vi "zad1.vi"() -> ()   [LabVIEW 2017]
panel:
  out "XY Graph":cluster{"Array":dbl[], dbl[]}(graph)
  out "error out":errorcluster
  in  "error in (no error)":errorcluster
  in  "Zakres":cluster{"Min":dbl, "Max":dbl, "Krok":dbl}
  in  "Wspo³czynniki wielomianu":cluster{"a":dbl, "b":dbl, "c":dbl, "d":dbl}
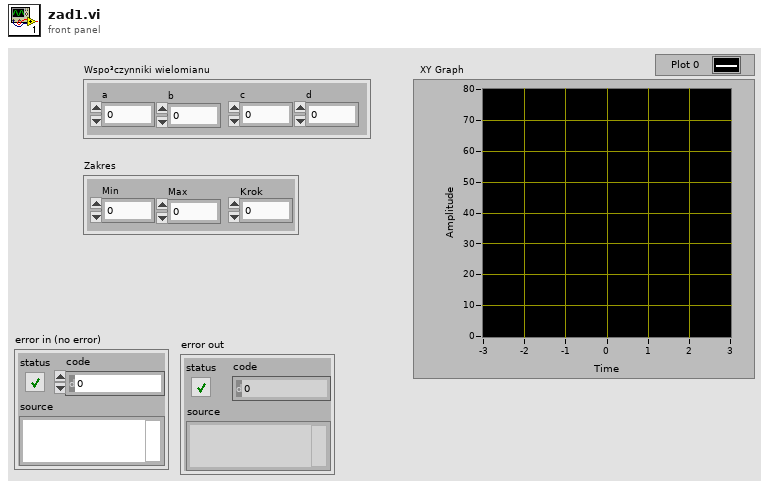
[diagram p1: front panel]
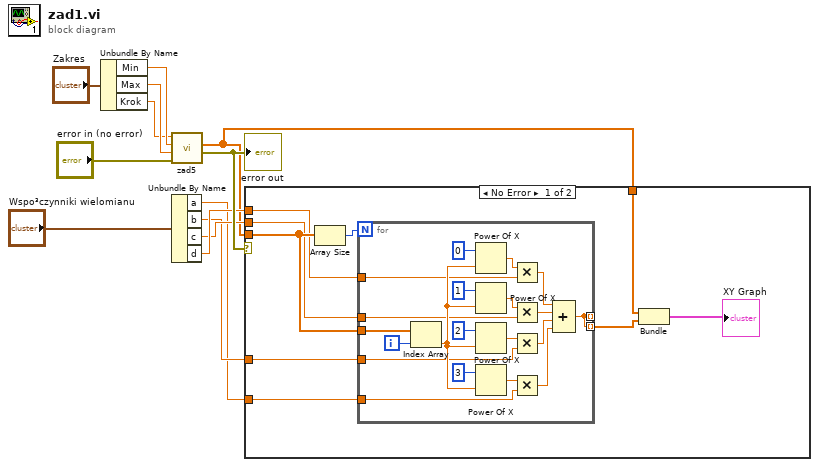
[diagram p0: block diagram]
diagram:
  n1 = Unbundle By Name("Zakres") -> ("Min"=w10:dbl, "Max"=w9:dbl, "Krok"=w8:dbl)
  n2 = call "zad5.vi"("error in (no error)"="error in (no error)", "Max"=w9, "Min"=w10, "Delta"=w8) -> ("error out"=w6:errorcluster, "Array"=w1:dbl[])  [unwired: 6 in]
  "error out" <- w6
  n3 = Unbundle By Name("Wspo³czynniki wielomianu") -> ("a"=w2:dbl, "b"=w3:dbl, "c"=w4:dbl, "d"=w5:dbl)
  n4 = case shown="No Error" w6 {
    tunnel: w1 -> [w21 _]
    tunnel: w5 -> [w20 _]
    tunnel: w4 -> [w19 _]
    tunnel: w3 -> [w18 _]
    tunnel: w2 -> [w17 _]
    tunnel: w1 -> [w14 _]
    frame No Error {
      n5 = Array Size(array=w21) -> (size(s)=w16:i32)
      n6 = for {
        N: w16 -> [_]
        tunnel: w21 -> [w41]
        tunnel: w20 -> [w38]
        tunnel: w19 -> [w34]
        tunnel: w18 -> [w33]
        tunnel: w17 -> [w32]
        tunnel: [w22] -> _ mode=indexing
        tunnel: [w22] -> w13 mode=indexing
        i -> [w27]
        n7 = Index Array(array=w41, index=w27) -> (element=w40:dbl)
        n8 = Power Of X(1:w40, 2:0) -> (0:w39:dbl)
        n9 = Power Of X(1:w40, 2:1) -> (0:w37:dbl)
        n10 = Power Of X(1:w40, 2:2) -> (0:w36:dbl)
        n11 = Power Of X(1:w40, 2:3) -> (0:w35:dbl)
        n12 = Multiply(x=w39, y=w38) -> (x*y=w31:dbl)
        n13 = Multiply(x=w37, y=w34) -> (x*y=w30:dbl)
        n14 = Multiply(x=w36, y=w33) -> (x*y=w29:dbl)
        n15 = Multiply(x=w35, y=w32) -> (x*y=w28:dbl)
        n16 = Compound Arithmetic op=ADD(w31, w30, w29, w28) -> (w22:dbl)
      }
      n17 = Bundle("Array"=w14, w13) -> (→"XY Graph":cluster{"Array":dbl[], dbl[]})  [unwired: 1 in]
    }
    frame Error {
    }
  }
